vi "Movie_ticket_booking_system.vi"() -> ()   [LabVIEW 2014]
uses:
  <vilib>/Utility/file.llb/Read From Spreadsheet File (I64).vi
  <vilib>/Utility/file.llb/Write To Spreadsheet File (I64).vi
panel:
  in  "back 2":bool
  in  "back":bool
  out "Choosen movie":i32=-1
  out "Movie4 file path":path
  out "first row 4":i64[](array[numeric])
  out "Movie3 file path":path
  out "first row 3":i64[](array[numeric])
  out "Movie2 file path":path
  out "first row 2":i64[](array[numeric])=[12, 13, 20, 21, 28, 29, 36, 37]
  out "first row 1":i64[](array[numeric])=[4, 5, 12, 19, 20, 27, 28, 36, 44, 45]
  out "Movie1 file path":path
  out "Consume time":i32
  out "Password":string
  out "Username":string
  out "login status":bool
  out "State":T1(ring)=enum."start"
  in  "Movie choose":T2
  in  "Register?":cluster{"OK Button 2":bool, "OK Button 3":bool}
  in  "Member?":cluster{"OK Button 2":bool, "OK Button 3":bool}
  in  "stop":bool
  in  "Start":bool
  out "String":string="Thank you for your custom!\nYou can leave or start a new booking!"
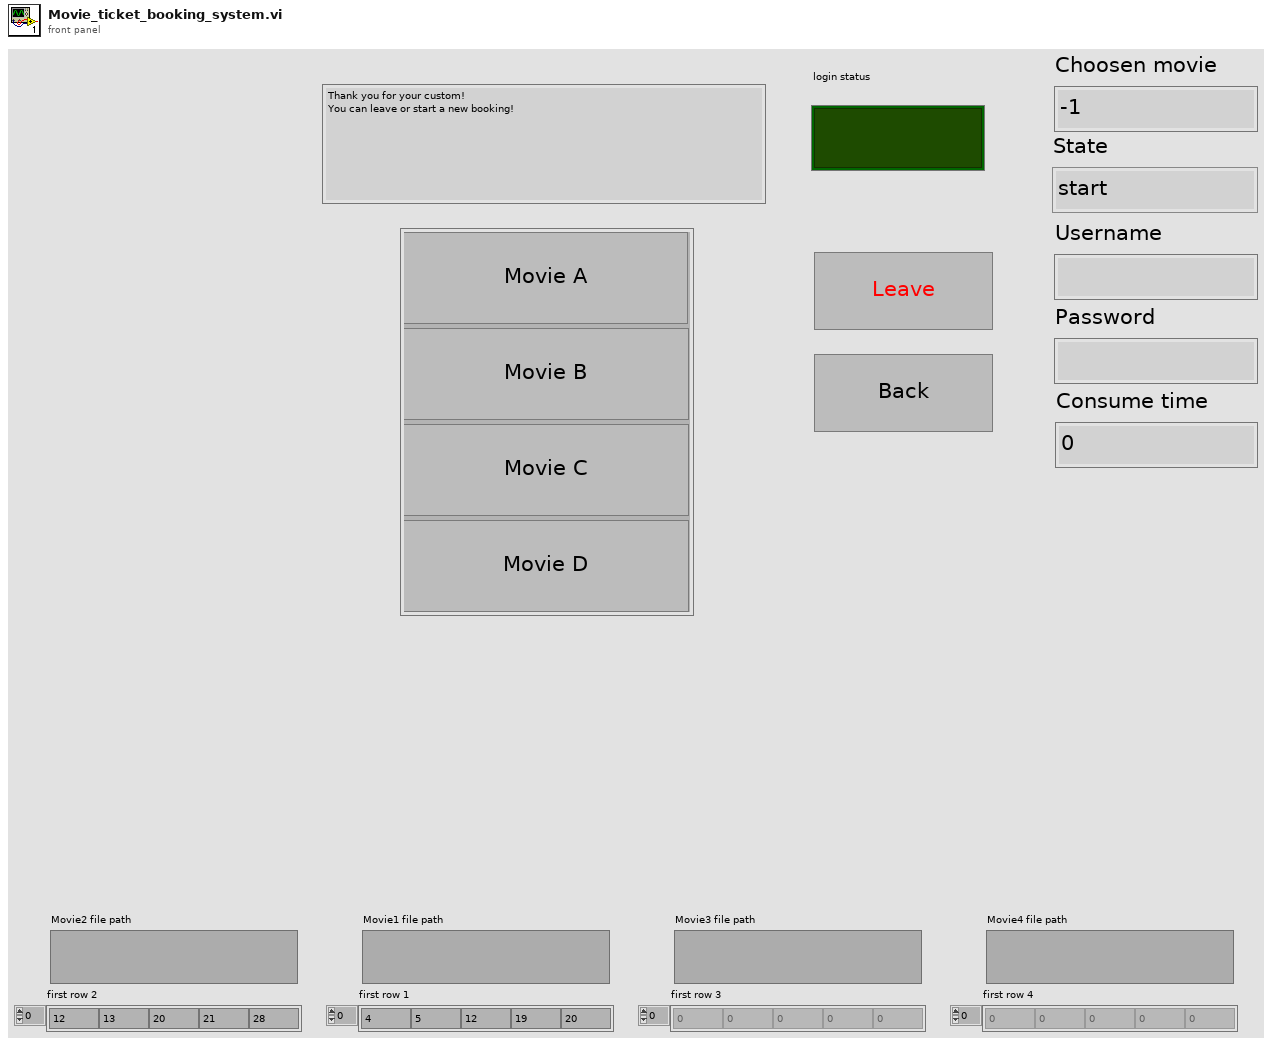
[diagram p1: front panel]
types:
  T1 = enum16{"initial", "start", "member?", "register?", "member login", "member register", "choose movie", "how many seat?", "check", "end"}
  T2 = cluster{"OK Button 3":bool, "OK Button 2":bool, "OK Button 4":bool, "OK Button 5":bool}
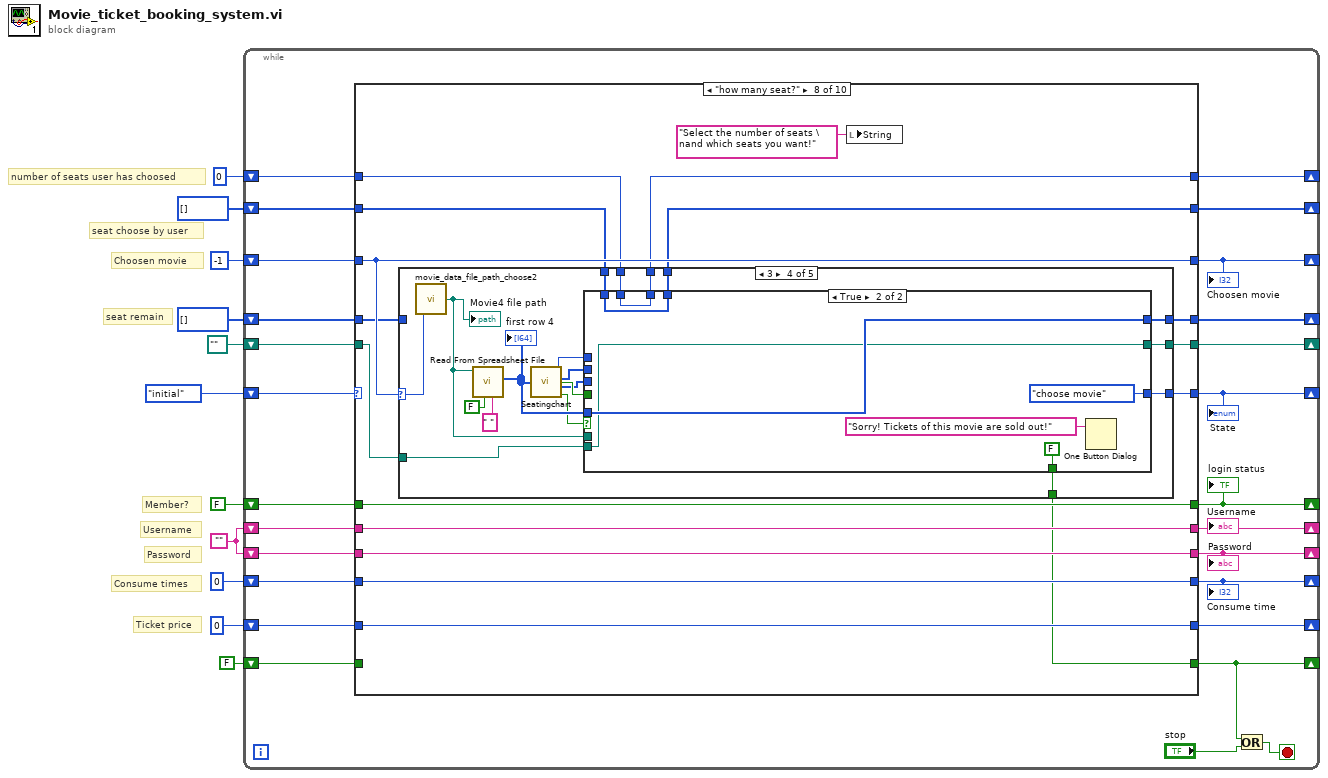
[diagram p0: block diagram]
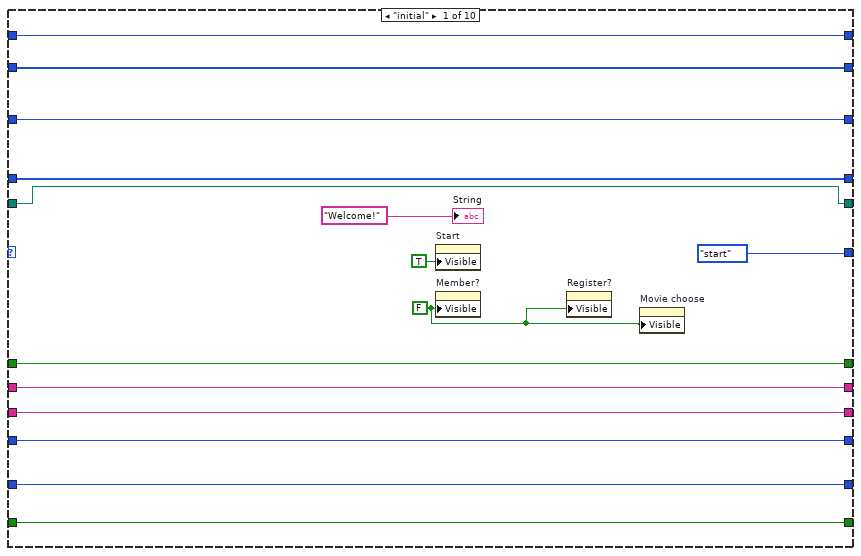
[diagram p2: hidden frame]
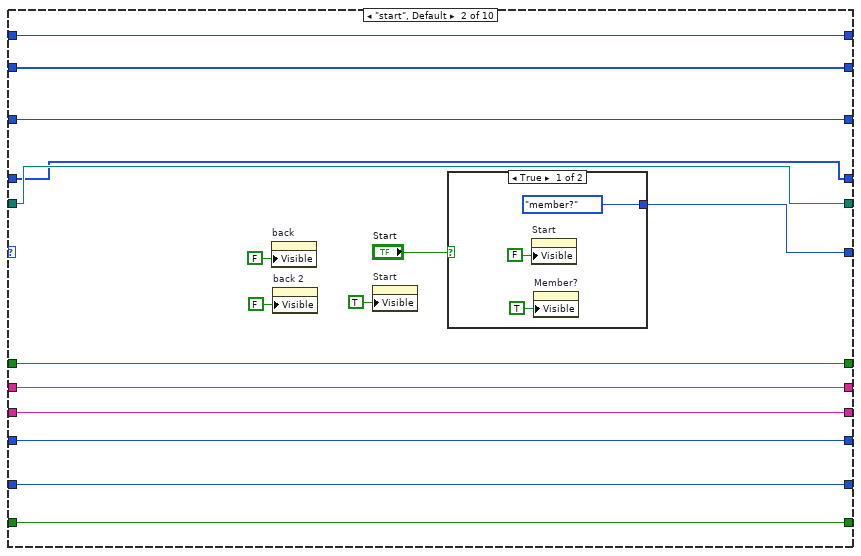
[diagram p3: hidden frame]
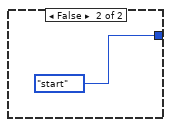
[diagram p4: hidden frame]
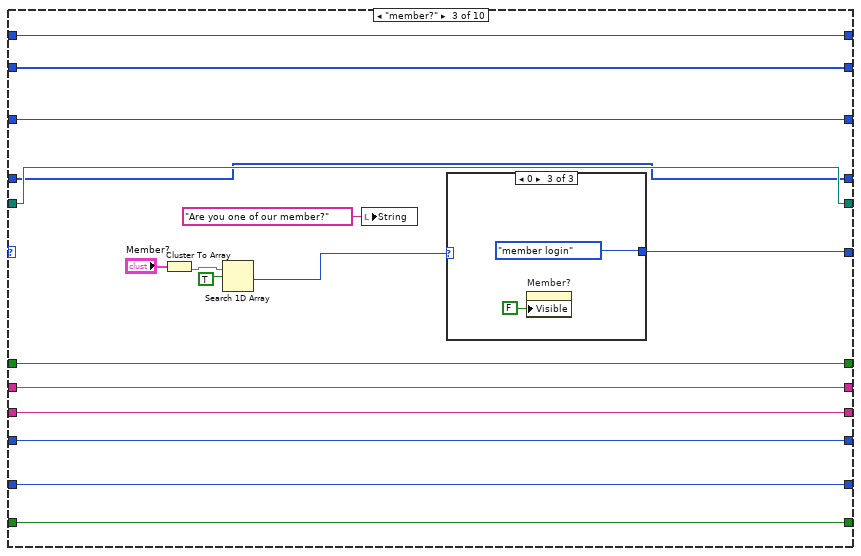
[diagram p5: hidden frame]
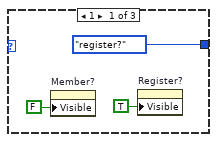
[diagram p6: hidden frame]
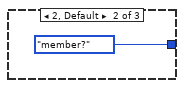
[diagram p7: hidden frame]
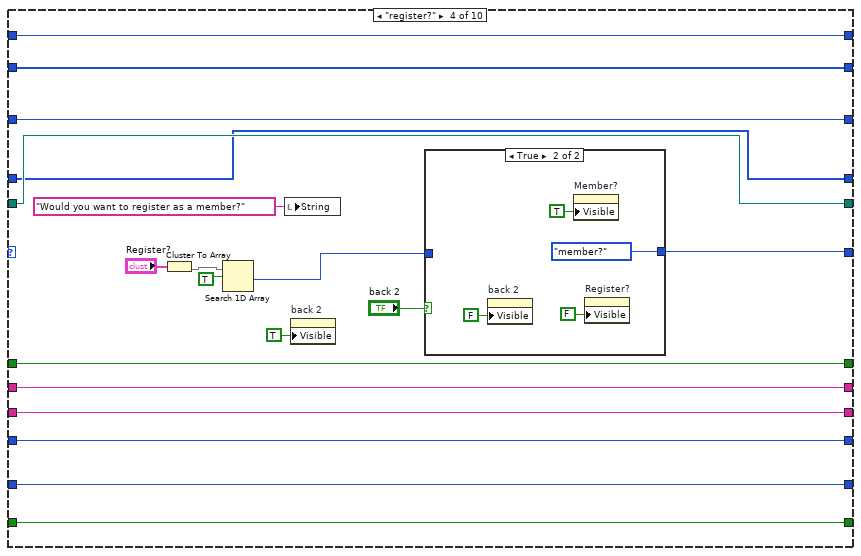
[diagram p8: hidden frame]
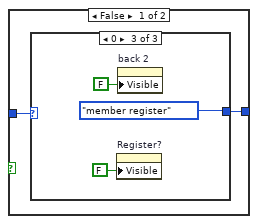
[diagram p9: hidden frame]
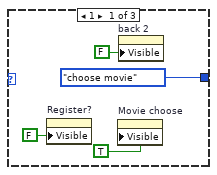
[diagram p10: hidden frame]
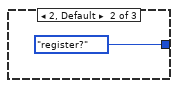
[diagram p11: hidden frame]
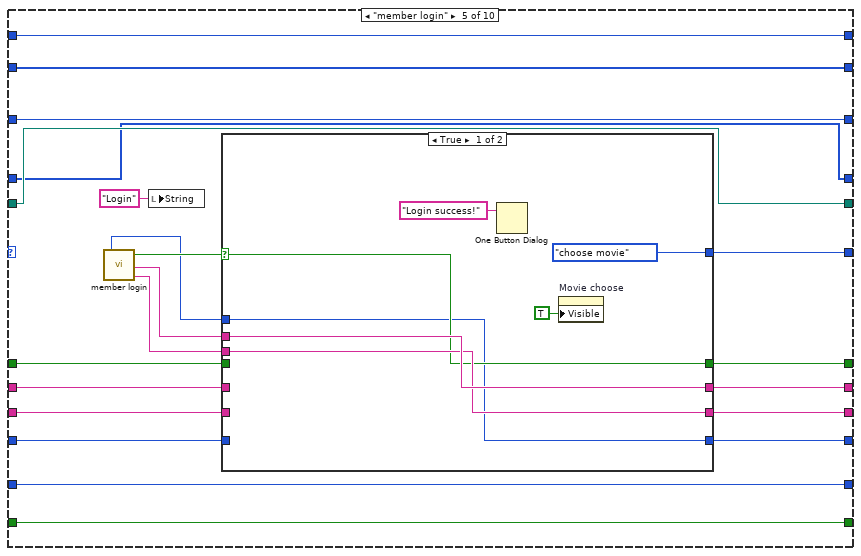
[diagram p12: hidden frame]
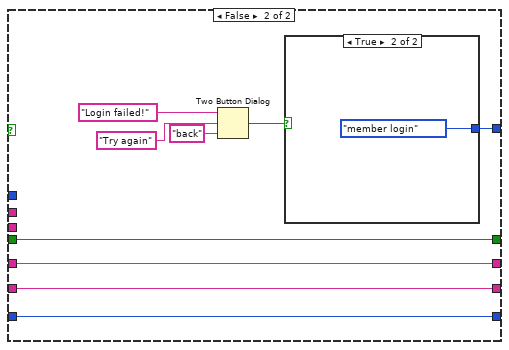
[diagram p13: hidden frame]
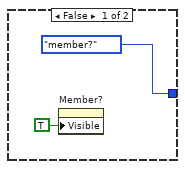
[diagram p14: hidden frame]
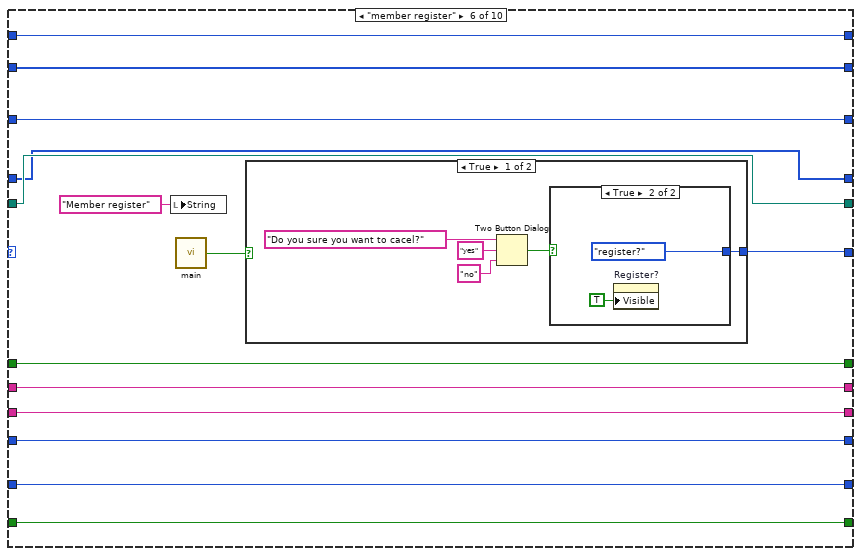
[diagram p15: hidden frame]
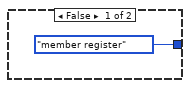
[diagram p16: hidden frame]
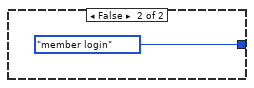
[diagram p17: hidden frame]
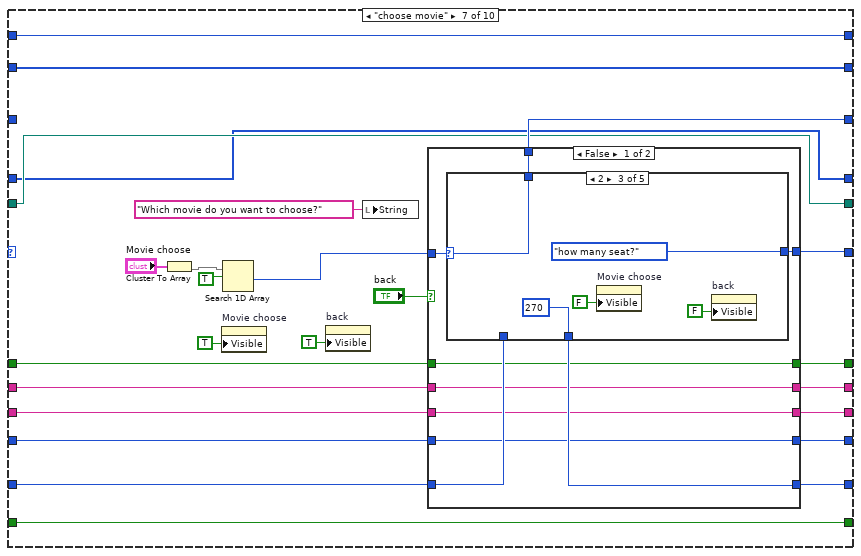
[diagram p18: hidden frame]
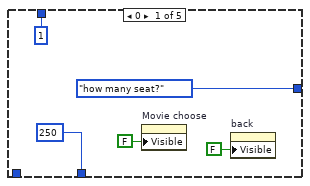
[diagram p19: hidden frame]
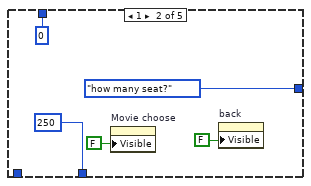
[diagram p20: hidden frame]
diagram:
  w10 = ""
  # "number of seats user has choosed"
  # "seat remain"
  # "seat choose by user"
  # "Ticket price"
  # "Choosen movie"
  # "Consume times"
  # "Member?"
  # "Password"
  # "Username"
  n1 = while {
    shift-right: [w36] -> _
    shift-left: T1."initial" -> [w37]
    shift-right: [w33] -> _
    shift-left: w10 -> [w35]
    shift-right: [w32] -> _
    shift-left: w10 -> [w34]
    shift-right: [w31] -> _
    shift-left: FALSE -> [w30]
    shift-right: [w29] -> _
    shift-left: 0 ("Numeric") -> [w28]
    shift-right: [w27] -> _
    shift-left: -1 ("index of element") -> [w26]
    shift-right: [w25] -> _
    shift-left: 0 ("No. of seats choosen") -> [w23]
    shift-right: [w24] -> _
    shift-left: i32[] [] -> [w22]
    shift-right: [w20] -> _
    shift-left: 0 -> [w21]
    shift-right: [w19] -> _
    shift-left: i64[] [] -> [w16]
    shift-right: [w18] -> _
    shift-left: path "" ("Movie4 file path") -> [w17]
    shift-right: [w13] -> _
    shift-left: FALSE ("Leave") -> [w15]
    stop <- w14 stop-if-true
    n2 = case shown="\"how many seat?\"" w37 {
      tunnel: [T1."start" w67 w84 w109 w148 w181 w211 w273 w507 w585] -> w36
      tunnel: w35 -> [w49 w66 w83 w108 w142 w180 w195 w272 w511 w597]
      tunnel: w34 -> [w48 w65 w82 w107 w141 w179 w196 w271 w520 w596]
      tunnel: [w49 w66 w83 w108 w144 w180 w194 w272 w510 w588] -> w33
      tunnel: [w48 w65 w82 w107 w143 w179 w197 w271 w520 w587] -> w32
      tunnel: [w47 w64 w81 w106 w140 w178 w193 w270 w509 w589] -> w31
      tunnel: w30 -> [w47 w64 w81 w106 w139 w178 w192 w270 w508 w598]
      tunnel: [w45 w63 w80 w105 w137 w176 w198 w269 w512 w586] -> w29
      tunnel: w28 -> [w45 w63 w80 w105 w136 w176 w199 w269 w513 w595]
      tunnel: [w44 w62 w79 w104 w135 w175 w210 w268 w501 w592] -> w27
      tunnel: w26 -> [w44 w62 w79 w104 w135 w175 _ w268 w502 w592]
      tunnel: [w42 w60 w77 w102 w133 w173 w207 w267 w498 w590] -> w25
      tunnel: [w43 w61 w78 w103 w134 w174 w208 w266 w499 w591] -> w24
      tunnel: w23 -> [w42 w60 w77 w102 w133 w173 w207 w265 w497 w590]
      tunnel: w22 -> [w43 w61 w78 w103 w134 w174 w208 w264 w500 w591]
      tunnel: w21 -> [w41 w58 w76 w101 w132 w172 w206 w263 w514 w584]
      tunnel: [w41 w58 w76 w101 w132 w172 w205 w263 w515 w584] -> w20
      tunnel: [w39 w56 w74 w99 w130 w170 w203 w262 w504 w593] -> w19
      tunnel: [w40 w57 w75 w100 w131 w171 w204 w261 w506 w594] -> w18
      tunnel: w17 -> [w40 w57 w75 w100 w131 w171 w204 w260 w505 w594]
      tunnel: w16 -> [w39 w56 w74 w99 w130 w170 w203 w259 w503 w593]
      tunnel: [w38 w55 w73 w98 w129 w169 w202 w258 w494 w583] -> w13
      tunnel: w15 -> [w38 w55 w73 w98 w129 w169 w202 _ _ w583]
      frame "initial" {
        w46 = FALSE ("Visible")
        n3 = property on="Start" class="Bool"("Visible"=TRUE) -> ()  [unwired: 2 in, 2 out]
        n4 = property on="Member?" class="Clust"("Visible"=w46) -> ()  [unwired: 2 in, 2 out]
        n5 = property on="Register?" class="Clust"("Visible"=w46) -> ()  [unwired: 2 in, 2 out]
        n6 = property on="Movie choose" class="Clust"("Visible"=w46) -> ()  [unwired: 2 in, 2 out]
        "String" <- "Welcome!" ("String")
      }
      frame "start", Default {
        n7 = property on="back" class="Bool"("Visible"=FALSE) -> ()  [unwired: 2 in, 2 out]
        n8 = property on="back 2" class="Bool"("Visible"=FALSE) -> ()  [unwired: 2 in, 2 out]
        n9 = property on="Start" class="Bool"("Visible"=TRUE) -> ()  [unwired: 2 in, 2 out]
        n10 = case shown="True" "Start" {
          tunnel: [T1."member?" T1."start"] -> w67
          frame True {
            n11 = property on="Start" class="Bool"("Visible"=FALSE) -> ()  [unwired: 2 in, 2 out]
            n12 = property on="Member?" class="Clust"("Visible"=TRUE) -> ()  [unwired: 2 in, 2 out]
          }
          frame False {
          }
        }
      }
      frame "member?" {
        n13 = Cluster To Array(cluster="Member?") -> (array=w87:bool[])
        n14 = Search 1D Array(1D array=w87, element=TRUE) -> (index of element=w85:i32)  [unwired: 1 in]
        n15 = local write "String"("Are you one of our member?" ("String")) -> ()
        n16 = case shown="0" w85 {
          tunnel: [T1."register?" T1."member?" T1."member login"] -> w84
          frame 1 {
            n17 = property on="Member?" class="Clust"("Visible"=FALSE) -> ()  [unwired: 2 in, 2 out]
            n18 = property on="Register?" class="Clust"("Visible"=TRUE) -> ()  [unwired: 2 in, 2 out]
          }
          frame 2, Default {
          }
          frame 0 {
            n19 = property on="Member?" class="Clust"("Visible"=FALSE) -> ()  [unwired: 2 in, 2 out]
          }
        }
      }
      frame "register?" {
        n20 = Cluster To Array(cluster="Register?") -> (array=w112:bool[])
        n21 = Search 1D Array(1D array=w112, element=TRUE) -> (index of element=w110:i32)  [unwired: 1 in]
        n22 = local write "String"("Would you want to register as a member?" ("String")) -> ()
        n23 = property on="back 2" class="Bool"("Visible"=TRUE) -> ()  [unwired: 2 in, 2 out]
        n24 = case shown="True" "back 2" {
          tunnel: w110 -> [w116 _]
          tunnel: [w115 T1."member?"] -> w109
          frame False {
            n25 = case shown="0" w116 {
              tunnel: [T1."choose movie" T1."register?" T1."member register"] -> w115
              frame 1 {
                n26 = property on="Register?" class="Clust"("Visible"=FALSE) -> ()  [unwired: 2 in, 2 out]
                n27 = property on="Movie choose" class="Clust"("Visible"=TRUE) -> ()  [unwired: 2 in, 2 out]
                n28 = property on="back 2" class="Bool"("Visible"=FALSE) -> ()  [unwired: 2 in, 2 out]
              }
              frame 2, Default {
              }
              frame 0 {
                n29 = property on="Register?" class="Clust"("Visible"=FALSE) -> ()  [unwired: 2 in, 2 out]
                n30 = property on="back 2" class="Bool"("Visible"=FALSE) -> ()  [unwired: 2 in, 2 out]
              }
            }
          }
          frame True {
            n31 = property on="back 2" class="Bool"("Visible"=FALSE) -> ()  [unwired: 2 in, 2 out]
            n32 = property on="Member?" class="Clust"("Visible"=TRUE) -> ()  [unwired: 2 in, 2 out]
            n33 = property on="Register?" class="Clust"("Visible"=FALSE) -> ()  [unwired: 2 in, 2 out]
          }
        }
      }
      frame "member login" {
        n34 = call "member login.vi"() -> ("Numeric"=w138:i32, "Pass?"=w147:bool, "Username"=w146:string, "Password"=w145:string)
        n35 = local write "String"("Login" ("String")) -> ()
        n36 = case shown="True" w147 {
          selector: w147 -> [w154 _]
          tunnel: [T1."choose movie" w159] -> w148
          tunnel: w146 -> [w156 _]
          tunnel: w145 -> [w155 _]
          tunnel: [w156 w165] -> w144
          tunnel: [w155 w164] -> w143
          tunnel: w142 -> [_ w165]
          tunnel: w141 -> [_ w164]
          tunnel: [w154 w158] -> w140
          tunnel: w139 -> [_ w158]
          tunnel: w138 -> [w151 _]
          tunnel: [w151 w157] -> w137
          tunnel: w136 -> [_ w157]
          frame True {
            n37 = One Button Dialog(message="Login success!") -> ()  [unwired: 1 in, 1 out]
            n38 = property on="Movie choose" class="Clust"("Visible"=TRUE) -> ()  [unwired: 2 in, 2 out]
          }
          frame False {
            n39 = Two Button Dialog(message="Login failed!", 1:"back" ("F button name (\"Cancel\")"), 2:"Try again" ("T button name (\"OK\")")) -> (T button?=w160:bool)
            n40 = case shown="True" w160 {
              tunnel: [T1."member?" T1."member login"] -> w159
              frame False {
                n41 = property on="Member?" class="Clust"("Visible"=TRUE) -> ()  [unwired: 2 in, 2 out]
              }
              frame True {
              }
            }
          }
        }
      }
      frame "member register" {
        n42 = local write "String"("Member register" ("String")) -> ()
        n43 = call "main.vi"() -> ("Cancel"=w177:bool)
        n44 = case shown="True" w177 {
          tunnel: [w183 T1."member login"] -> w181
          frame True {
            n45 = Two Button Dialog(message="Do you sure you want to cacel?", 1:"no" ("F button name (\"Cancel\")"), 2:"yes" ("T button name (\"OK\")")) -> (T button?=w187:bool)
            n46 = case shown="True" w187 {
              tunnel: [T1."member register" T1."register?"] -> w183
              frame False {
              }
              frame True {
                n47 = property on="Register?" class="Clust"("Visible"=TRUE) -> ()  [unwired: 2 in, 2 out]
              }
            }
          }
          frame False {
          }
        }
      }
      frame "choose movie" {
        n48 = Cluster To Array(cluster="Movie choose") -> (array=w214:bool[])
        n49 = property on="Movie choose" class="Clust"("Visible"=TRUE) -> ()  [unwired: 2 in, 2 out]
        n50 = Search 1D Array(1D array=w214, element=TRUE) -> (index of element=w212:i32)  [unwired: 1 in]
        n51 = property on="back" class="Bool"("Visible"=TRUE) -> ()  [unwired: 2 in, 2 out]
        n52 = local write "String"("Which movie do you want to choose?" ("String")) -> ()
        n53 = case shown="False" "back" {
          tunnel: w212 -> [w225 _]
          tunnel: [w224 T1."member?"] -> w211
          tunnel: [w223 -1] -> w210
          tunnel: w206 -> [w222 w255]
          tunnel: [w221 w255] -> w205
          tunnel: w199 -> [w220 _]
          tunnel: [w220 0 ("Numeric")] -> w198
          tunnel: [w219 w250] -> w197
          tunnel: w196 -> [w219 _]
          tunnel: w195 -> [w218 _]
          tunnel: [w218 w250] -> w194
          tunnel: [w217 FALSE] -> w193
          tunnel: w192 -> [w217 _]
          frame False {
            n54 = case shown="2" w225 {
              selector: w225 -> [_ _ w238 w243 _]
              tunnel: [T1."how many seat?" T1."how many seat?" T1."how many seat?" T1."how many seat?" T1."choose movie"] -> w224
              tunnel: [1 ("index of element") 0 ("index of element") w238 w243 -1] -> w223
              tunnel: w222 -> [_ _ _ _ w246]
              tunnel: [250 250 270 300 w246] -> w221
              frame 0 {
                n55 = property on="Movie choose" class="Clust"("Visible"=FALSE) -> ()  [unwired: 2 in, 2 out]
                n56 = property on="back" class="Bool"("Visible"=FALSE) -> ()  [unwired: 2 in, 2 out]
              }
              frame 1 {
                n57 = property on="Movie choose" class="Clust"("Visible"=FALSE) -> ()  [unwired: 2 in, 2 out]
                n58 = property on="back" class="Bool"("Visible"=FALSE) -> ()  [unwired: 2 in, 2 out]
              }
              frame 2 {
                n59 = property on="Movie choose" class="Clust"("Visible"=FALSE) -> ()  [unwired: 2 in, 2 out]
                n60 = property on="back" class="Bool"("Visible"=FALSE) -> ()  [unwired: 2 in, 2 out]
              }
              frame 3 {
                n61 = property on="Movie choose" class="Clust"("Visible"=FALSE) -> ()  [unwired: 2 in, 2 out]
                n62 = property on="back" class="Bool"("Visible"=FALSE) -> ()  [unwired: 2 in, 2 out]
              }
              frame 4, Default {
              }
            }
          }
          frame True {
            w250 = ""
            n63 = property on="Member?" class="Clust"("Visible"=TRUE) -> ()  [unwired: 2 in, 2 out]
            n64 = property on="Movie choose" class="Clust"("Visible"=FALSE) -> ()  [unwired: 2 in, 2 out]
            n65 = property on="back" class="Bool"("Visible"=FALSE) -> ()  [unwired: 2 in, 2 out]
          }
        }
      }
      frame "how many seat?" {
        n66 = case shown="3" w268 {
          selector: w268 -> [w276 w329 w382 w435 _]
          tunnel: [w287 w340 w393 w446 T1."how many seat?"] -> w273
          tunnel: [w286 w339 w392 w445 w493] -> w267
          tunnel: [w285 w338 w391 w444 w492] -> w266
          tunnel: w265 -> [w284 w337 w390 w443 w493]
          tunnel: w264 -> [w283 w336 w389 w442 w492]
          tunnel: [w282 w335 w388 w441 w488] -> w262
          tunnel: [w280 w334 w387 w440 w489] -> w261
          tunnel: w260 -> [w279 w332 w385 w439 w489]
          tunnel: w259 -> [_ _ _ _ w488]
          tunnel: [w278 w331 w384 w437 FALSE ("Leave")] -> w258
          frame 0 {
            n67 = call "movie_data_file_path_choose2.vi"("CM"=w276) -> ("appended path"=w277:path)
            "Movie1 file path" <- w277
            n68 = call-poly <vilib>:"Read From Spreadsheet File.vi"("delimiter (\\t)"=" " ("delimiter (\\t)"), "transpose (no:F)"=FALSE, "file path (dialog if empty)"=w277) -> ("first row"=w281:i64[])  [unwired: 4 in, 4 out]
            "first row 1" <- w281
            n69 = call "Seatingchart.vi"("selected seats before"=w281) -> ("No seat"=w275:bool, "selected seats after"=w290:i32[], "seats selected by user"=w289:i32[], "No. of seats choosen"=w288:i32, "Cancel"=w291:bool)
            n70 = case shown="True" w275 {
              tunnel: w291 -> [w308 _]
              tunnel: w290 -> [w307 _]
              tunnel: w289 -> [w306 _]
              tunnel: w288 -> [w305 _]
              tunnel: [w304 T1."choose movie" ("Next state")] -> w287
              tunnel: [w303 w322] -> w286
              tunnel: [w302 w321] -> w285
              tunnel: w284 -> [w301 w322]
              tunnel: w283 -> [w300 w321]
              tunnel: [w299 w324] -> w282
              tunnel: w281 -> [w298 w324]
              tunnel: [w297 w325] -> w280
              tunnel: w279 -> [w296 w325]
              tunnel: [w295 FALSE ("Leave")] -> w278
              tunnel: w277 -> [w294 _]
              frame False {
                n71 = case shown="False" w308 {
                  tunnel: w307 -> [w311 _]
                  tunnel: w306 -> [w312 _]
                  tunnel: w305 -> [w313 _]
                  tunnel: [T1."check" w320] -> w304
                  tunnel: w294 -> [w310 _]
                  tunnel: [w313 w319] -> w303
                  tunnel: [w312 w318] -> w302
                  tunnel: w301 -> [_ w319]
                  tunnel: w300 -> [_ w318]
                  tunnel: [w311 w317] -> w299
                  tunnel: w298 -> [_ w317]
                  tunnel: [w310 w316] -> w297
                  tunnel: w296 -> [_ w316]
                  tunnel: [FALSE ("Leave") w315] -> w295
                  frame False {
                  }
                  frame True {
                    n72 = call "what_do_you_want.vi"() -> ("Next state"=w320:T1, "Leave"=w315:bool)
                  }
                }
              }
              frame True {
                n73 = One Button Dialog(message="Sorry! Tickets of this movie are sold out!") -> ()  [unwired: 1 in, 1 out]
              }
            }
          }
          frame 1 {
            n74 = call "movie_data_file_path_choose2.vi"("CM"=w329) -> ("appended path"=w330:path)
            "Movie2 file path" <- w330
            n75 = call-poly <vilib>:"Read From Spreadsheet File.vi"("delimiter (\\t)"=" " ("delimiter (\\t)"), "transpose (no:F)"=FALSE, "file path (dialog if empty)"=w330) -> ("first row"=w333:i64[])  [unwired: 4 in, 4 out]
            "first row 2" <- w333
            n76 = call "Seatingchart.vi"("selected seats before"=w333) -> ("No seat"=w328:bool, "selected seats after"=w343:i32[], "seats selected by user"=w342:i32[], "No. of seats choosen"=w341:i32, "Cancel"=w344:bool)
            n77 = case shown="True" w328 {
              tunnel: w344 -> [w361 _]
              tunnel: w343 -> [w360 _]
              tunnel: w342 -> [w359 _]
              tunnel: w341 -> [w358 _]
              tunnel: [w357 T1."choose movie" ("Next state")] -> w340
              tunnel: [w356 w375] -> w339
              tunnel: [w355 w374] -> w338
              tunnel: w337 -> [w354 w375]
              tunnel: w336 -> [w353 w374]
              tunnel: [w352 w378] -> w335
              tunnel: [w351 w379] -> w334
              tunnel: w333 -> [w350 w378]
              tunnel: w332 -> [w349 w379]
              tunnel: [w348 FALSE ("Leave")] -> w331
              tunnel: w330 -> [w347 _]
              frame False {
                n78 = case shown="False" w361 {
                  tunnel: w360 -> [w364 _]
                  tunnel: w359 -> [w365 _]
                  tunnel: w358 -> [w366 _]
                  tunnel: [T1."check" w373] -> w357
                  tunnel: w347 -> [w363 _]
                  tunnel: [w366 w372] -> w356
                  tunnel: [w365 w371] -> w355
                  tunnel: w354 -> [_ w372]
                  tunnel: w353 -> [_ w371]
                  tunnel: [w364 w370] -> w352
                  tunnel: [w363 w369] -> w351
                  tunnel: w350 -> [_ w370]
                  tunnel: w349 -> [_ w369]
                  tunnel: [FALSE ("Leave") w368] -> w348
                  frame False {
                  }
                  frame True {
                    n79 = call "what_do_you_want.vi"() -> ("Next state"=w373:T1, "Leave"=w368:bool)
                  }
                }
              }
              frame True {
                n80 = One Button Dialog(message="Sorry! Tickets of this movie are sold out!") -> ()  [unwired: 1 in, 1 out]
              }
            }
          }
          frame 2 {
            n81 = call "movie_data_file_path_choose2.vi"("CM"=w382) -> ("appended path"=w383:path)
            "Movie3 file path" <- w383
            n82 = call-poly <vilib>:"Read From Spreadsheet File.vi"("delimiter (\\t)"=" " ("delimiter (\\t)"), "transpose (no:F)"=FALSE, "file path (dialog if empty)"=w383) -> ("first row"=w386:i64[])  [unwired: 4 in, 4 out]
            "first row 3" <- w386
            n83 = call "Seatingchart.vi"("selected seats before"=w386) -> ("No seat"=w381:bool, "selected seats after"=w396:i32[], "seats selected by user"=w395:i32[], "No. of seats choosen"=w394:i32, "Cancel"=w397:bool)
            n84 = case shown="True" w381 {
              tunnel: w397 -> [w414 _]
              tunnel: w396 -> [w413 _]
              tunnel: w395 -> [w412 _]
              tunnel: w394 -> [w411 _]
              tunnel: [w410 T1."choose movie" ("Next state")] -> w393
              tunnel: [w409 w430] -> w392
              tunnel: [w408 w429] -> w391
              tunnel: w390 -> [w407 w430]
              tunnel: w389 -> [w406 w429]
              tunnel: [w405 w428] -> w388
              tunnel: [w404 w427] -> w387
              tunnel: w386 -> [w403 w428]
              tunnel: w385 -> [w402 w427]
              tunnel: [w401 FALSE] -> w384
              tunnel: w383 -> [w400 _]
              frame False {
                n85 = case shown="True" w414 {
                  tunnel: w413 -> [w417 _]
                  tunnel: w412 -> [w418 _]
                  tunnel: w411 -> [w419 _]
                  tunnel: [T1."check" w426] -> w410
                  tunnel: w400 -> [w416 _]
                  tunnel: [w419 w425] -> w409
                  tunnel: [w418 w424] -> w408
                  tunnel: w407 -> [_ w425]
                  tunnel: w406 -> [_ w424]
                  tunnel: [w417 w423] -> w405
                  tunnel: [w416 w422] -> w404
                  tunnel: w403 -> [_ w423]
                  tunnel: w402 -> [_ w422]
                  tunnel: [FALSE ("Leave") w421] -> w401
                  frame False {
                  }
                  frame True {
                    n86 = call "what_do_you_want.vi"() -> ("Next state"=w426:T1, "Leave"=w421:bool)
                  }
                }
              }
              frame True {
                n87 = One Button Dialog(message="Sorry! Tickets of this movie are sold out!") -> ()  [unwired: 1 in, 1 out]
              }
            }
          }
          frame 3 {
            n88 = call "movie_data_file_path_choose2.vi"("CM"=w435) -> ("appended path"=w436:path)
            "Movie4 file path" <- w436
            n89 = call-poly <vilib>:"Read From Spreadsheet File.vi"("delimiter (\\t)"=" " ("delimiter (\\t)"), "transpose (no:F)"=FALSE, "file path (dialog if empty)"=w436) -> ("first row"=w438:i64[])  [unwired: 4 in, 4 out]
            "first row 4" <- w438
            n90 = call "Seatingchart.vi"("selected seats before"=w438) -> ("No seat"=w434:bool, "selected seats after"=w449:i32[], "seats selected by user"=w448:i32[], "No. of seats choosen"=w447:i32, "Cancel"=w450:bool)
            n91 = case shown="True" w434 {
              tunnel: w450 -> [w467 _]
              tunnel: w449 -> [w466 _]
              tunnel: w448 -> [w465 _]
              tunnel: w447 -> [w464 _]
              tunnel: [w463 T1."choose movie" ("Next state")] -> w446
              tunnel: [w462 w481] -> w445
              tunnel: [w461 w480] -> w444
              tunnel: w443 -> [w460 w481]
              tunnel: w442 -> [w459 w480]
              tunnel: [w458 w483] -> w441
              tunnel: [w457 w482] -> w440
              tunnel: w439 -> [w456 w482]
              tunnel: w438 -> [w455 w483]
              tunnel: [w454 FALSE ("Leave")] -> w437
              tunnel: w436 -> [w453 _]
              frame False {
                n92 = case shown="False" w467 {
                  tunnel: w466 -> [w470 _]
                  tunnel: w465 -> [w471 _]
                  tunnel: w464 -> [w472 _]
                  tunnel: [T1."check" w479] -> w463
                  tunnel: w453 -> [w469 _]
                  tunnel: [w472 w478] -> w462
                  tunnel: [w471 w477] -> w461
                  tunnel: w460 -> [_ w478]
                  tunnel: w459 -> [_ w477]
                  tunnel: [w470 w475] -> w458
                  tunnel: [w469 w476] -> w457
                  tunnel: w456 -> [_ w476]
                  tunnel: w455 -> [_ w475]
                  tunnel: [FALSE ("Leave") w474] -> w454
                  frame False {
                  }
                  frame True {
                    n93 = call "what_do_you_want.vi"() -> ("Next state"=w479:T1, "Leave"=w474:bool)
                  }
                }
              }
              frame True {
                n94 = One Button Dialog(message="Sorry! Tickets of this movie are sold out!") -> ()  [unwired: 1 in, 1 out]
              }
            }
          }
          frame 4, Default {
            n95 = One Button Dialog(message="Perhap something is wrong!") -> ()  [unwired: 1 in, 1 out]
          }
        }
        n96 = local write "String"("Select the number of seats \nand which seats you want!" ("String")) -> ()
      }
      frame "check" {
        n97 = call "check_comfirm.vi"("Choose movie"=w502, "NOC"=w513, "No. of seats"=w497, "Price"=w514, "Username"=w511, "member"=w508, "Seats no."=w500) -> ("finish check"=w518:bool, "Next state"=w517:T1, "TA"=w516:dbl, "Leave"=w495:bool)
        n98 = case shown="True" w518 {
          tunnel: w517 -> [w526 _]
          tunnel: w516 -> [_ w553]
          tunnel: [0 w550] -> w515
          tunnel: w514 -> [_ w549]
          tunnel: w513 -> [w529 w548]
          tunnel: [w529 w547] -> w512
          tunnel: w511 -> [w528 w546]
          tunnel: [w528 w545] -> w510
          tunnel: [w527 w544] -> w509
          tunnel: w508 -> [w527 w543]
          tunnel: [w526 w542] -> w507
          tunnel: [path "" ("Movie4 file path") w541] -> w506
          tunnel: w505 -> [_ w540]
          tunnel: [w524 w539] -> w504
          tunnel: w503 -> [_ w538]
          tunnel: w502 -> [_ w537]
          tunnel: [-1 ("index of element") w536] -> w501
          tunnel: w500 -> [_ w535]
          tunnel: [w524 w534] -> w499
          tunnel: [0 ("No. of seats choosen") w532] -> w498
          tunnel: w497 -> [_ w533]
          tunnel: [FALSE w531] -> w496
          frame False {
            w524 = i32[] []
          }
          frame True {
            n99 = call "paying.vi"("Total Amount(In)"=w553) -> ("Boolean"=w552:bool, "Next state"=w551:T1, "Leave"=w531:bool)
            n100 = case shown="False" w552 {
              tunnel: w551 -> [_ w578]
              tunnel: [0 0] -> w550
              tunnel: w549 -> [_ _]
              tunnel: w548 -> [w565 w581]
              tunnel: [w559 w581] -> w547
              tunnel: w546 -> [w563 w580]
              tunnel: [w563 w580] -> w545
              tunnel: w543 -> [w554 w579]
              tunnel: [w554 w579] -> w544
              tunnel: [T1."end" ("Next state") w578] -> w542
              tunnel: w540 -> [w566 _]
              tunnel: [path "" ("Movie4 file path") path "" ("Movie4 file path")] -> w541
              tunnel: w538 -> [w567 _]
              tunnel: [w562 w575] -> w539
              tunnel: w537 -> [_ _]
              tunnel: [-1 ("index of element") -1 ("index of element")] -> w536
              tunnel: w535 -> [_ _]
              tunnel: [w562 w575] -> w534
              tunnel: w533 -> [w558 _]
              tunnel: [0 ("No. of seats choosen") 0 ("No. of seats choosen")] -> w532
              frame False {
                w562 = i32[] []
                n101 = case shown="False" w554 {
                  tunnel: w565 -> [w569 w572]
                  tunnel: [w569 w571] -> w559
                  tunnel: w558 -> [_ w570]
                  frame False {
                  }
                  frame True {
                    n102 = Add(x=w570, y=w572) -> (x+y=w571:i32)
                  }
                }
                n103 = call-poly <vilib>:"Write To Spreadsheet File.vi"("delimiter (\\t)"=" " ("delimiter (\\t)"), "transpose? (no:F)"=FALSE, "1D data"=w567, "file path (dialog if empty)"=w566) -> ()  [unwired: 4 in, 1 out]
              }
              frame True {
                w575 = i32[] []
              }
            }
          }
        }
        n104 = Or(x=w496, y=w495) -> (x .or. y?=w494:bool)
        n105 = local write "String"("Please check your booking information and pay the bill!" ("String")) -> ()
      }
      frame "end" {
        n106 = case shown="True" w598 {
          selector: w598 -> [w602 w612]
          tunnel: w597 -> [w601 w605]
          tunnel: w596 -> [w600 w611]
          tunnel: w595 -> [w599 w604]
          tunnel: [w602 w610] -> w589
          tunnel: [w601 w609] -> w588
          tunnel: [w600 w608] -> w587
          tunnel: [w599 w607] -> w586
          tunnel: [T1."start" w606] -> w585
          frame False {
          }
          frame True {
            n107 = call "member_data_save.vi"("NOC"=w604, "Username"=w605) -> ()
            n108 = call "what_do_you_want_end.vi"() -> ("Log out"=w613:bool)
            n109 = case shown="True" w613 {
              tunnel: w605 -> [w617 _]
              tunnel: w604 -> [w615 _]
              tunnel: w612 -> [w618 _]
              tunnel: w611 -> [w616 _]
              tunnel: [w618 FALSE] -> w610
              tunnel: [w617 w621] -> w609
              tunnel: [w616 w621] -> w608
              tunnel: [w615 0 ("Numeric")] -> w607
              tunnel: [T1."choose movie" T1."start"] -> w606
              frame False {
              }
              frame True {
                w621 = ""
              }
            }
          }
        }
        n110 = local write "String"("Thank you for your custom!\nYou can leave or start a new booking!" ("String")) -> ()
      }
    }
    "State" <- w36
    "login status" <- w31
    "Username" <- w33
    "Password" <- w32
    "Consume time" <- w29
    "Choosen movie" <- w27
    n111 = Or(x=w13, y="stop") -> (x .or. y?=w14:bool)
  }
